vi "Windspeed Warnings.vi"() -> ()   [LabVIEW 2017]
uses:
  Weather Data.ctl
panel:
  out "Weather Data Out":T1={"Current Temperature"=0.0, "Max Temperature"=0.0, "Min Temperature"=0.0, "Warning?"=FALSE, "Warning Text"="No Warning", "Units"=enum."Celcius", "Current Windspeed"=0.0, "Max Windspeed"=0.0, "Windspeed Warning?"=FALSE, "Windspeed Warning Text"="No Warning"}
  in  "Weather Data In":T1={"Current Temperature"=0.0, "Max Temperature"=0.0, "Min Temperature"=0.0, "Warning?"=FALSE, "Warning Text"="No Warning", "Units"=enum."Celcius", "Current Windspeed"=0.0, "Max Windspeed"=0.0, "Windspeed Warning?"=FALSE, "Windspeed Warning Text"="No Warning"}
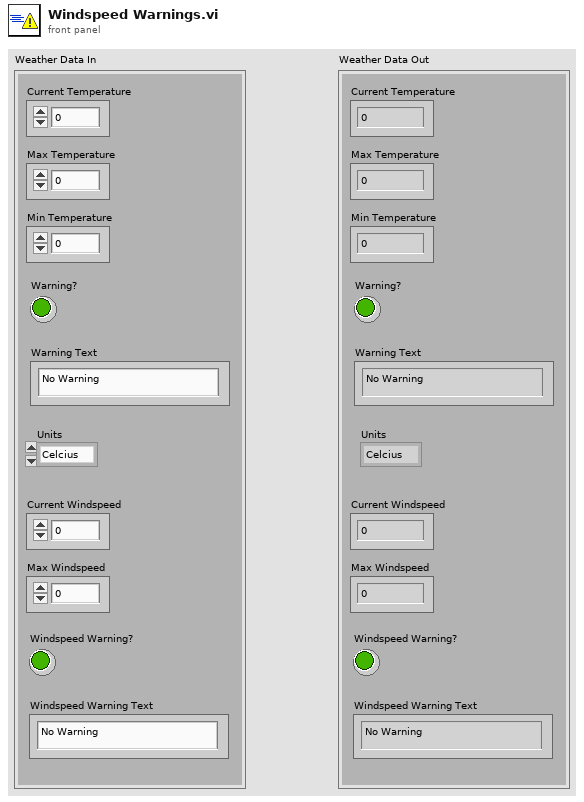
[diagram p1: front panel]
types:
  T1 = typedef "Weather Data.ctl" = cluster{"Current Temperature":dbl, "Max Temperature":dbl, "Min Temperature":dbl, "Warning?":bool, "Warning Text":string, "Units":enum16{"Celcius", "Farenheit"}, "Current Windspeed":dbl, "Max Windspeed":dbl, "Windspeed Warning?":bool, "Windspeed Warning Text":string}
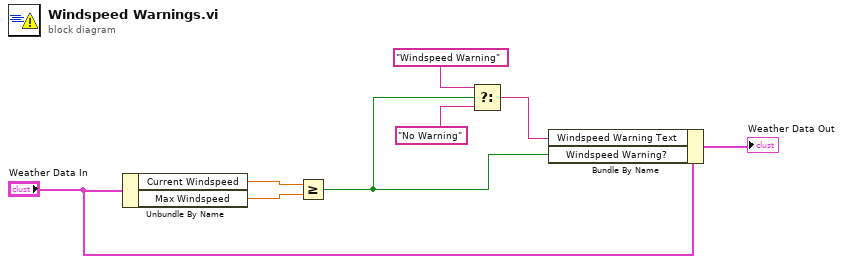
[diagram p0: block diagram]
diagram:
  n1 = Unbundle By Name("Weather Data In") -> ("Current Windspeed"=w6:dbl, "Max Windspeed"=w5:dbl)
  n2 = Greater Or Equal?(x=w6, y=w5) -> (x >= y?=w2:bool)
  n3 = Select(t="Windspeed Warning", s=w2, f="No Warning") -> (s? t:f=w1:string)
  n4 = Bundle By Name(cluster="Weather Data In", "Windspeed Warning Text"=w1, "Windspeed Warning?"=w2) -> (→"Weather Data Out":T1)
